vi "LR700 Select Sensor.vi"(2 "Parameters":dbl[](array[numeric]) format="%.3e", 3 "Instrument Address":refnum<visa-resource-name>) -> (0 "Stop":bool, 1 "Array":dbl[](array[numeric]) format="%.2f")   [LabVIEW 2021]
doc: "This VI reads the AVS resistance bridge.\nScott Hannahs, NHMFL-FSU, Nov 1993"
panel:
  # "First parameter is the sensor number\nSecond parameter is the wait in seconds"
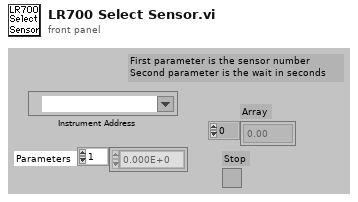
[diagram p1: front panel]
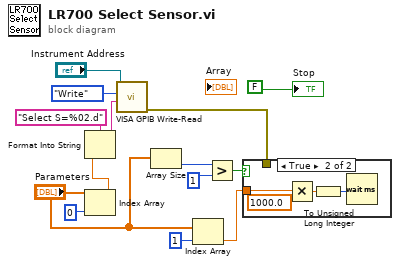
[diagram p0: block diagram]
diagram:
  n1 = Index Array(array="Parameters", index=0) -> (element=w12:dbl)
  n2 = Format Into String(format string="Select S=%02.d", w12) -> (resulting string=w9:string)  [unwired: 2 in, 1 out]
  n3 = call "VISA GPIB Write-Read.vi"("Command"=w9, "Action"=enum16{"Write", "Read", "Write & Read"}."Write", "VISA resource name"="Instrument Address") -> ("error out"=w8:errorcluster)  [unwired: 5 in, 3 out]
  n4 = Array Size(array="Parameters") -> (size(s)=w6:i32)
  n5 = Index Array(array="Parameters", index=1) -> (element=w11:dbl)
  n6 = Greater?(x=w6, y=1) -> (0:w4:bool)
  n7 = case shown="True" w4 {
    tunnel: w11 -> [_ w17]
    tunnel: w8 -> [_ _]
    frame False {
    }
    frame True {
      n8 = Multiply(x=w17, y=1000.0) -> (x*y=w16:dbl)
      n9 = To Unsigned Long Integer(number=w16) -> (unsigned 32bit integer=w15:u32)
      n10 = Wait (ms)(milliseconds to wait=w15) -> ()  [unwired: 1 out]
    }
  }
  "Stop" <- FALSE
